vi "dataset.create_commit.vi"(8 "error in":errorcluster, 11 "DatasetCreateStaging in":refnum<class "DatasetCreateStaging.lvclass">) -> (0 "error out":errorcluster, 2 "Dataset":refnum<class "Dataset.lvclass">, 3 "DatasetCreateStaging out":refnum<class "DatasetCreateStaging.lvclass">)   [LabVIEW 2020, in "DatasetCreateStaging.lvclass"]
doc: "Creates the staged dataset in Nominal and returns a handle to it."
uses:
  DatasetCreateStaging.lvclass
  Dataset/Dataset.lvclass
  DatasetCreateStaging.lvclass/DatasetCreateStaging.ctl
  Dataset/Dataset.lvclass/Dataset.ctl
  client.lvlib
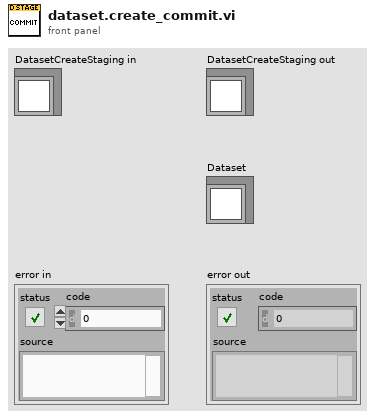
[diagram p1: front panel]
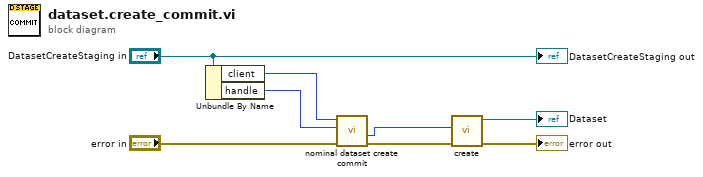
[diagram p0: block diagram]
diagram:
  n1 = Unbundle By Name("DatasetCreateStaging in") -> ("client"=w7:i32, "handle"=w5:i32)
  n2 = call "nominal dataset create commit.vi"("error in (no error)"="error in", "staging"=w5, "client"=w7) -> ("error out"=w1:errorcluster, "out_dataset out"=w4:i32)  [unwired: 6 in, 1 out]
  n3 = call "create.vi"("error in (no error)"=w1, "handle"=w4) -> ("error out"=→"error out":errorcluster, "Dataset out"=→"Dataset":refnum<class "Dataset.lvclass">)  [unwired: 8 in]
  "DatasetCreateStaging out" <- "DatasetCreateStaging in"
